vi "Czujnik pradu.vi"() -> ()   [LabVIEW 2019]
panel:
  out "XY Graph":cluster{dbl[], dbl[]}[](graph)
  in  "Array -75A":dbl[](array[numeric])=[2.50768, 2.48474, 2.45196, 2.42543, 2.39573, 2.37772, 2.22753, 2.08658, 1.94639]
  in  "Array 75A":dbl[](array[numeric])=[2.5134, 2.54237, 2.57356, 2.60176, 2.62721, 2.6568, 2.79527, 2.93786, 3.08438]
  in  "Array -35A":dbl[](array[numeric])=[2.51031, 2.44668, 2.38002, 2.31258, 2.2474, 2.18325, 1.84899, 1.50553, 1.16945]
  in  "Array 35A":dbl[](array[numeric])=[2.52112, 2.59097, 2.66381, 2.72137, 2.78988, 2.85665, 3.19265, 3.52993, 3.87006]
  in  "Array -5A":dbl[](array[numeric])=[2.55242, 2.36032, 2.18287, 2.0016, 1.81906, 1.62978]
  in  "Array 5A":dbl[](array[numeric])=[2.55635, 2.73186, 2.9154, 3.09798, 3.29916, 3.45912]
  # "0,1,2,3,4,5,10,15,20"
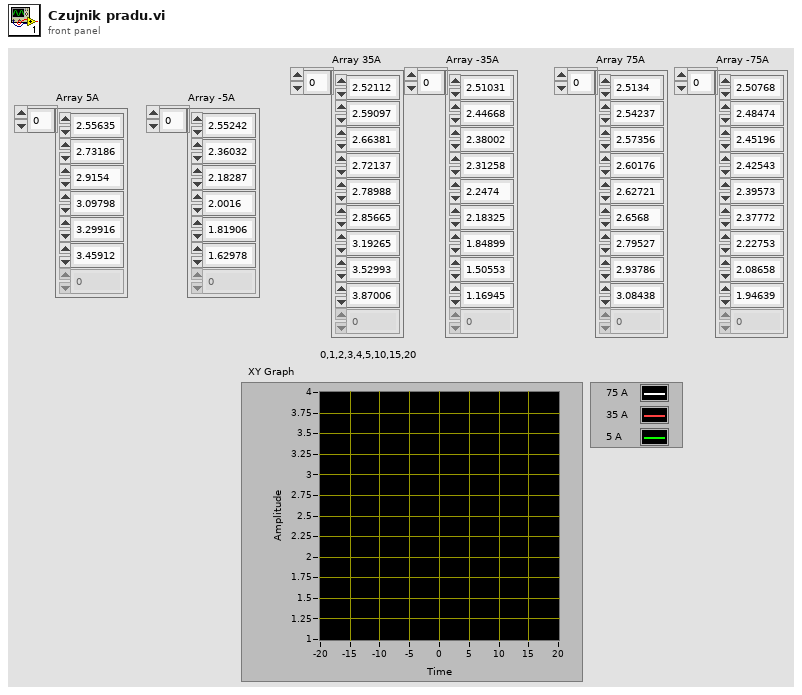
[diagram p1: front panel]
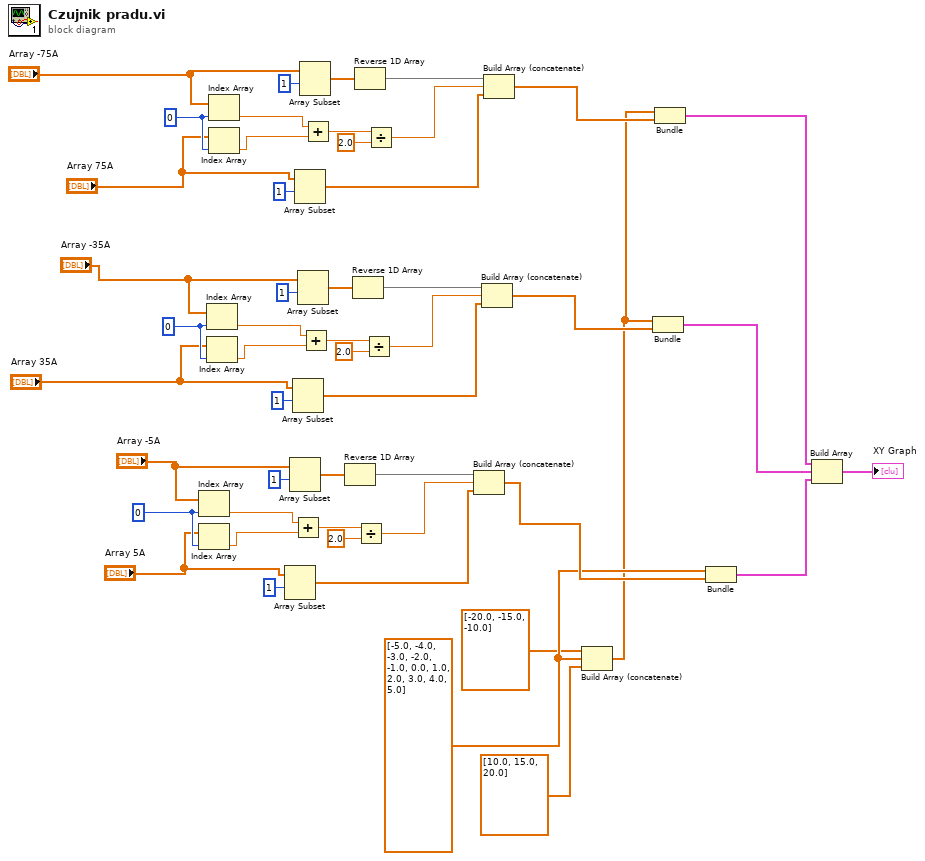
[diagram p0: block diagram]
diagram:
  w18 = 0 ("index")
  w23 = 0 ("index")
  w36 = dbl[] [-5.0, -4.0, -3.0, -2.0, -1.0, 0.0, 1.0, 2.0, 3.0, 4.0, 5.0]
  w50 = 0 ("index")
  n1 = Index Array(array="Array -5A", index=w50) -> (element=w42:dbl)
  n2 = Index Array(array="Array 5A", index=w50) -> (element=w41:dbl)
  n3 = Index Array(array="Array -35A", index=w23) -> (element=w29:dbl)
  n4 = Index Array(array="Array 35A", index=w23) -> (element=w30:dbl)
  n5 = Index Array(array="Array -75A", index=w18) -> (element=w12:dbl)
  n6 = Index Array(array="Array 75A", index=w18) -> (element=w11:dbl)
  n7 = Array Subset(array="Array 5A", index=1) -> (w43:dbl[])  [unwired: 1 in]
  n8 = Array Subset(array="Array -5A", index=1) -> (w47:dbl[])  [unwired: 1 in]
  n9 = Array Subset(array="Array 35A", index=1) -> (w28:dbl[])  [unwired: 1 in]
  n10 = Add(x=w42, y=w41) -> (x+y=w40:dbl)
  n11 = Array Subset(array="Array 75A", index=1) -> (w13:dbl[])  [unwired: 1 in]
  n12 = Array Subset(array="Array -35A", index=1) -> (w25:dbl[])  [unwired: 1 in]
  n13 = Array Subset(array="Array -75A", index=1) -> (w16:dbl[])  [unwired: 1 in]
  n14 = Add(x=w29, y=w30) -> (x+y=w31:dbl)
  n15 = Add(x=w12, y=w11) -> (x+y=w10:dbl)
  n16 = Reverse 1D Array(array=w47) -> (reversed array=w44:dbl[])
  n17 = Reverse 1D Array(array=w25) -> (reversed array=w27:dbl[])
  n18 = Reverse 1D Array(array=w16) -> (reversed array=w14:dbl[])
  n19 = Divide(x=w40, y=2.0) -> (x/y=w38:dbl)
  n20 = Divide(x=w31, y=2.0) -> (x/y=w33:dbl)
  n21 = Divide(x=w10, y=2.0) -> (x/y=w8:dbl)
  n22 = Build Array (concatenate)(w44, w38, w43) -> (w37:dbl[])
  n23 = Build Array (concatenate)(w27, w33, w28) -> (w22:dbl[])
  n24 = Build Array (concatenate)(w14, w8, w13) -> (w19:dbl[])
  n25 = Build Array (concatenate)(dbl[] [-20.0, -15.0, -10.0], w36, dbl[] [10.0, 15.0, 20.0]) -> (w5:dbl[])
  n26 = Bundle(w5, w22) -> (w3:cluster{dbl[], dbl[]})  [unwired: 1 in]
  n27 = Bundle(w5, w19) -> (w2:cluster{dbl[], dbl[]})  [unwired: 1 in]
  n28 = Bundle(w36, w37) -> (w4:cluster{dbl[], dbl[]})  [unwired: 1 in]
  n29 = Build Array(w2, w3, w4) -> (→"XY Graph":cluster{dbl[], dbl[]}[])
